vi "aft_Calc_FXP_Settings.vi"(0 "fixed-point configurations":T2) -> (1 "x":T1, 2 "d":T1, 3 "w":T1, 4 "init1":T1, 6 "init2":T1, 10 "init3":T1, 12 "cast 1":T1, 13 "cast 2":T1, 14 "step":T1, 15 "init4":T1)   [LabVIEW 2017, in "NI_AdaptiveFilter.lvlib"]
uses:
  <vilib>/addons/Adaptive Filters/NI_AdaptiveFilter.lvlib
  <vilib>/fxp/LVFixedPointRepBitsTypeDef.ctl
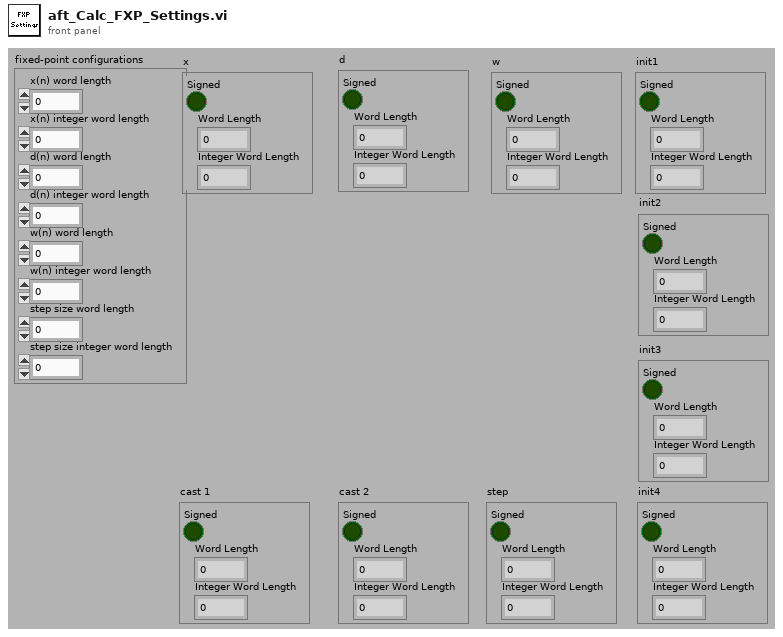
[diagram p1: front panel]
types:
  T1 = typedef "LVFixedPointRepBitsTypeDef.ctl" = cluster{"Signed":bool, "Word Length":u32, "Integer Word Length":i32}
  T2 = cluster{"x(n) word length":i32, "x(n) integer word length":i32, "d(n) word length":i32, "d(n) integer word length":i32, "w(n) word length":i32, "w(n) integer word length":i32, "step size word length":i32, "step size integer word length":i32}
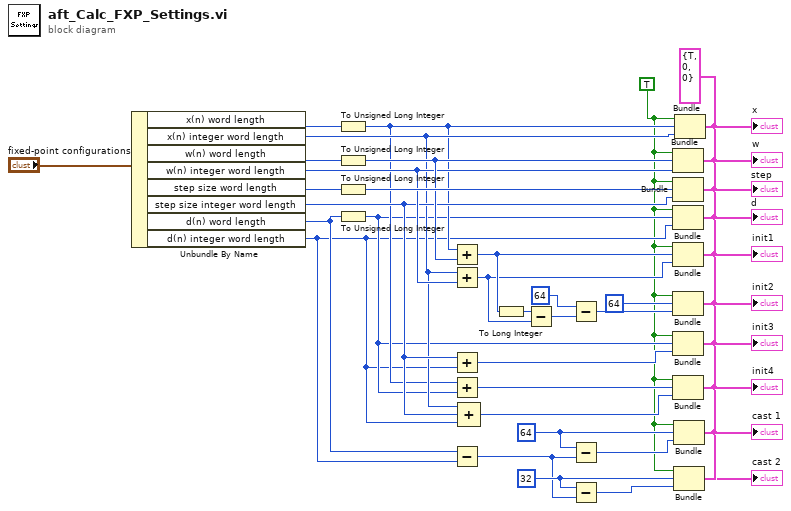
[diagram p0: block diagram]
diagram:
  w2 = 32
  w7 = 64
  w6 = T1 {"Signed"=TRUE, "Word Length"=0, "Integer Word Length"=0} ("x")
  w4 = TRUE
  n1 = Unbundle By Name("fixed-point configurations") -> ("x(n) word length"=w36:i32, "x(n) integer word length"=w26:i32, "w(n) word length"=w37:i32, "w(n) integer word length"=w34:i32, "step size word length"=w39:i32, "step size integer word length"=w27:i32, "d(n) word length"=w13:i32, "d(n) integer word length"=w12:i32)
  n2 = To Unsigned Long Integer(number=w36) -> (unsigned 32bit integer=w15:u32)
  n3 = To Unsigned Long Integer(number=w37) -> (unsigned 32bit integer=w35:u32)
  n4 = To Unsigned Long Integer(number=w39) -> (unsigned 32bit integer=w38:u32)
  n5 = To Unsigned Long Integer(number=w13) -> (unsigned 32bit integer=w14:u32)
  n6 = Add(x=w15, y=w35) -> (x+y=w33:u32)
  n7 = Add(x=w26, y=w34) -> (x+y=w32:i32)
  n8 = Add(x=w27, y=w12) -> (x+y=w28:i32)
  n9 = Add(x=w15, y=w14) -> (x+y=w25:u32)
  n10 = Subtract(x=w13, y=w12) -> (x-y=w1:i32)
  n11 = Compound Arithmetic op=ADD(w26, w27, w12) -> (w24:i32)
  n12 = To Long Integer(number=w33) -> (32bit integer=w29:i32)
  n13 = Subtract(x=w29, y=w32) -> (x-y=w31:i32)
  n14 = Subtract(x=64, y=w31) -> (x-y=w11:i32)
  n15 = Subtract(x=w7, y=w1) -> (x-y=w8:i32)
  n16 = Subtract(x=w2, y=w1) -> (x-y=w3:i32)
  n17 = Bundle(cluster=w6, "Signed"=w4, "Word Length"=w35, "Integer Word Length"=w34) -> (→"w":T1)
  n18 = Bundle(cluster=w6, "Signed"=w4, "Word Length"=w38, "Integer Word Length"=w27) -> (→"step":T1)
  n19 = Bundle(cluster=w6, "Signed"=w4, "Word Length"=w14, "Integer Word Length"=w12) -> (→"d":T1)
  n20 = Bundle(cluster=w6, "Signed"=w4, "Word Length"=w33, "Integer Word Length"=w32) -> (→"init1":T1)
  n21 = Bundle(cluster=w6, "Signed"=w4, "Word Length"=u32 64, "Integer Word Length"=w11) -> (→"init2":T1)
  n22 = Bundle(cluster=w6, "Signed"=w4, "Word Length"=w14, "Integer Word Length"=w28) -> (→"init3":T1)
  n23 = Bundle(cluster=w6, "Signed"=w4, "Word Length"=w25, "Integer Word Length"=w24) -> (→"init4":T1)
  n24 = Bundle(cluster=w6, "Signed"=w4, "Word Length"=w7, "Integer Word Length"=w8) -> (→"cast 1":T1)
  n25 = Bundle(cluster=w6, "Signed"=w4, "Word Length"=w2, "Integer Word Length"=w3) -> (→"cast 2":T1)
  n26 = Bundle(cluster=w6, "Signed"=w4, "Word Length"=w15, "Integer Word Length"=w26) -> (→"x":T1)
